vi "event structure data.vi"() -> ()   [LabVIEW 2016]
uses:
  <vilib>/measure/NI_MABase.lvlib
panel:
  in  "Plot color":u32(colorbox)
  in  "stop":bool
  out "Waveform Chart":waveform(dbl)(graph)
  in  "Amplitude":dbl(knob) scale=0.0..10.0
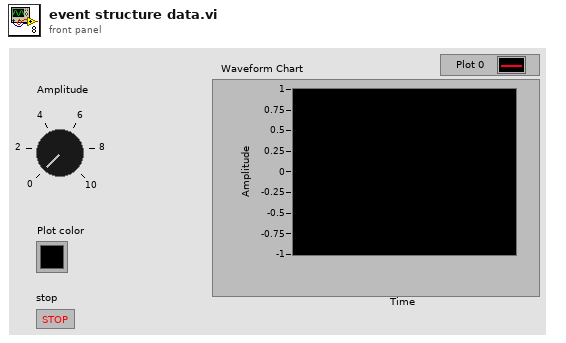
[diagram p1: front panel]
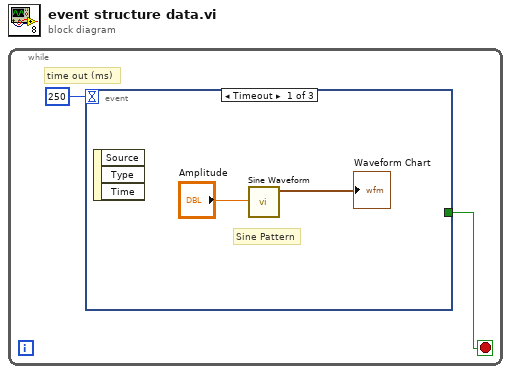
[diagram p0: block diagram]
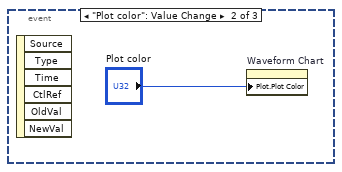
[diagram p2: hidden frame]
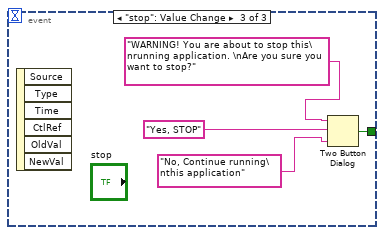
[diagram p3: hidden frame]
diagram:
  n1 = while {
    stop <- w1 stop-if-true
    # "time out (ms)"
    n2 = event shown="[0] Timeout" {
      selector: _ -> [_ _ _]
      dyn-events: _ -> [_ _ _]
      timeout: 250 -> [_ _ _]
      tunnel: [_ _ w6] -> w1
      event Timeout {
        # "Sine Pattern"
        n3 = event-data() -> ()  [unwired: 1 in, 3 out]
        n4 = call <vilib>:"Sine Waveform.vi"("amplitude"="Amplitude") -> ("signal out"=→"Waveform Chart":waveform(dbl))  [unwired: 9 in, 1 out]
      }
      event "Plot color": Value Change {
        n5 = event-data() -> ()  [unwired: 1 in, 6 out]
        n6 = property on="Waveform Chart" class="WFChart (strict)"("Plot.Plot Color"="Plot color") -> ()  [unwired: 2 in, 2 out]
      }
      event "stop": Value Change {
        n7 = event-data() -> ()  [unwired: 1 in, 6 out]
        n8 = Two Button Dialog(message="WARNING! You are about to stop this\nrunning application. \nAre you sure you want to stop?", 1:"No, Continue running\nthis application", 2:"Yes, STOP") -> (T button?=w6:bool)
      }
    }
  }
